vi "test_min-wpts.vi"() -> ()   [LabVIEW 2019]
uses:
  Ctrl/waypoint_buf.ctl
panel:
  in  "Tab Control":enum32{"Page 1", "ref"}(tab)
  out "XY Graph":cluster{cluster{dbl, dbl}[]}[](graph)=[{[{1.0, 2.0}]}, {[{1.0, 3.0}, {1.0980171403295607, 2.995184726672197}, {1.1950903220161282, 2.9807852804032304}, {1.2902846772544623, 2.9569403357322086}, {1.3826834323650898, 2.923879532511287}, {1.4713967368259977, 2.881921264348355}, {1.5555702330196022, 2.8314696123025453}, {1.6343932841636455, 2.773010453362737}, {1.7071067811865475, 2.7071067811865475}, {1.7730104533627369, 2.6343932841636457}, {1.8314696123025453, 2.555570233019602}, {1.881921264348355, 2.471396736825998}, {1.9238795325112867, 2.3826834323650896}, {1.956940335732209, 2.2902846772544625}, {1.9807852804032304, 2.1950903220161284}, {1.9951847266721967, 2.098017140329561}, {2.0, 2.0}, {1.995184726672197, 1.9019828596704393}, {1.9807852804032304, 1.8049096779838718}, {1.956940335732209, 1.709715322745538}, {1.9238795325112867, 1.6173165676349104}, {1.881921264348355, 1.5286032631740023}, {1.8314696123025453, 1.444429766980398}, {1.773010453362737, 1.3656067158363547}, {1.7071067811865475, 1.2928932188134525}, {1.6343932841636455, 1.2269895466372631}, {1.5555702330196022, 1.1685303876974547}, {1.471396736825998, 1.118078735651645}, {1.3826834323650898, 1.0761204674887133}, {1.2902846772544625, 1.0430596642677912}, {1.1950903220161286, 1.0192147195967696}, {1.0980171403295609, 1.0048152733278033}, {1.0000000000000002, 1.0}, {0.9019828596704395, 1.004815273327803}, {0.8049096779838716, 1.0192147195967696}, {0.709715322745538, 1.043059664267791}, {0.6173165676349104, 1.076120467488713}, {0.5286032631740023, 1.118078735651645}, {0.44442976698039804, 1.1685303876974547}, {0.36560671583635473, 1.226989546637263}, {0.29289321881345254, 1.2928932188134523}, {0.22698954663726334, 1.365606715836354}, {0.16853038769745476, 1.4444297669803978}, {0.11807873565164506, 1.528603263174002}, {0.07612046748871348, 1.6173165676349097}, {0.043059664267791176, 1.7097153227455375}, {0.01921471959676968, 1.8049096779838714}, {0.004815273327803071, 1.9019828596704396}, {0.0, 1.9999999999999998}, {0.004815273327803071, 2.09801714032956}, {0.01921471959676957, 2.1950903220161284}, {0.043059664267791065, 2.290284677254462}, {0.07612046748871337, 2.38268343236509}, {0.11807873565164495, 2.4713967368259975}, {0.16853038769745454, 2.5555702330196017}, {0.22698954663726312, 2.6343932841636457}, {0.2928932188134523, 2.7071067811865475}, {0.36560671583635407, 2.773010453362737}, {0.4444297669803978, 2.8314696123025453}, {0.5286032631740021, 2.881921264348355}, {0.6173165676349096, 2.9238795325112865}, {0.7097153227455375, 2.9569403357322086}, {0.8049096779838713, 2.9807852804032304}, {0.9019828596704395, 2.995184726672197}, {0.9999999999999998, 3.0}]}, {[{-1.0, 1.5}, {3.5, 3.0}, {5.0, 2.5}, {10.0, 4.0}, {13.0, 0.0}, {10.0, -3.0}, {5.0, -4.0}, {2.0, -3.0}, {-1.0, -5.0}, {-2.0, -2.0}, {-1.0, 1.0}]}, {[{-1.0, 1.5}, {-0.9042553191489362, 1.5319148936170213}, {-0.8085106382978724, 1.5638297872340425}, {-0.7127659574468085, 1.5957446808510638}, {-0.6170212765957447, 1.627659574468085}, {-0.5212765957446809, 1.6595744680851063}, {-0.42553191489361697, 1.6914893617021276}, {-0.32978723404255317, 1.7234042553191489}, {-0.23404255319148937, 1.7553191489361701}, {-0.13829787234042556, 1.7872340425531914}, {-0.042553191489361764, 1.8191489361702127}, {0.05319148936170204, 1.851063829787234}, {0.14893617021276606, 1.8829787234042552}, {0.24468085106382986, 1.9148936170212765}, {0.34042553191489366, 1.9468085106382977}, {0.43617021276595747, 1.978723404255319}, {0.5319148936170213, 2.0106382978723403}, {0.6276595744680851, 2.0425531914893615}, {0.7234042553191489, 2.074468085106383}, {0.8191489361702127, 2.106382978723404}, {0.9148936170212765, 2.1382978723404253}, {1.0106382978723403, 2.1702127659574466}, {1.106382978723404, 2.202127659574468}, {1.2021276595744679, 2.234042553191489}, {1.2978723404255321, 2.2659574468085104}, {1.393617021276596, 2.297872340425532}, {1.4893617021276597, 2.329787234042553}, {1.5851063829787235, 2.3617021276595747}, {1.6808510638297873, 2.3936170212765955}, {1.7765957446808511, 2.425531914893617}, {1.872340425531915, 2.457446808510638}, {1.9680851063829787, 2.4893617021276597}, {2.0638297872340425, 2.5212765957446805}, {2.1595744680851063, 2.5531914893617023}, {2.25531914893617, 2.585106382978723}, {2.351063829787234, 2.617021276595745}, {2.4468085106382977, 2.6489361702127656}, {2.5425531914893615, 2.6808510638297873}, {2.6382978723404253, 2.712765957446808}, {2.734042553191489, 2.74468085106383}, {2.829787234042553, 2.7765957446808507}, {2.925531914893617, 2.8085106382978724}, {3.0212765957446805, 2.840425531914893}, {3.117021276595745, 2.872340425531915}, {3.212765957446808, 2.9042553191489358}, {3.3085106382978724, 2.9361702127659575}, {3.4042553191489358, 2.9680851063829783}, {3.5, 3.0}, {3.59375, 2.96875}, {3.6875, 2.9375}, {3.78125, 2.90625}, {3.875, 2.875}, {3.96875, 2.84375}, {4.0625, 2.8125}, {4.15625, 2.78125}, {4.25, 2.75}, {4.34375, 2.71875}, {4.4375, 2.6875}, {4.53125, 2.65625}, {4.625, 2.625}, {4.71875, 2.59375}, {4.8125, 2.5625}, {4.90625, 2.53125}, {5.0, 2.5}, {5.096153846153846, 2.5288461538461537}, {5.1923076923076925, 2.5576923076923075}, {5.288461538461538, 2.5865384615384617}, {5.384615384615385, 2.6153846153846154}, {5.480769230769231, 2.644230769230769}, {5.576923076923077, 2.673076923076923}, {5.673076923076923, 2.701923076923077}, {5.769230769230769, 2.730769230769231}, {5.865384615384615, 2.7596153846153846}, {5.961538461538462, 2.7884615384615383}, {6.0576923076923075, 2.8173076923076925}, {6.153846153846154, 2.8461538461538463}, {6.25, 2.875}, {6.346153846153847, 2.9038461538461537}, {6.4423076923076925, 2.9326923076923075}, {6.538461538461538, 2.9615384615384617}, {6.634615384615385, 2.9903846153846154}, {6.730769230769231, 3.019230769230769}, {6.826923076923077, 3.0480769230769234}, {6.923076923076923, 3.076923076923077}, {7.019230769230769, 3.105769230769231}, {7.115384615384615, 3.1346153846153846}, {7.211538461538462, 3.1634615384615383}, {7.307692307692308, 3.1923076923076925}, {7.403846153846154, 3.2211538461538463}, {7.5, 3.25}, {7.596153846153847, 3.2788461538461537}, {7.6923076923076925, 3.3076923076923075}, {7.788461538461538, 3.3365384615384617}, {7.884615384615385, 3.3653846153846154}, {7.980769230769231, 3.394230769230769}, {8.076923076923077, 3.4230769230769234}, {8.173076923076923, 3.451923076923077}, {8.26923076923077, 3.480769230769231}, {8.365384615384615, 3.5096153846153846}, {8.461538461538462, 3.5384615384615383}, {8.557692307692308, 3.5673076923076925}, {8.653846153846153, 3.5961538461538463}, {8.75, 3.625}, {8.846153846153847, 3.653846153846154}, {8.942307692307693, 3.6826923076923075}, {9.038461538461538, 3.7115384615384617}, {9.134615384615385, 3.7403846153846154}, {9.23076923076923, 3.769230769230769}, {9.326923076923077, 3.7980769230769234}, {9.423076923076923, 3.826923076923077}, {9.51923076923077, 3.855769230769231}, {9.615384615384617, 3.8846153846153846}, {9.711538461538462, 3.9134615384615383}, {9.807692307692308, 3.9423076923076925}, {9.903846153846153, 3.9711538461538463}, {10.0, 4.0}, {10.06, 3.92}, {10.12, 3.84}, {10.18, 3.76}, {10.24, 3.68}, {10.3, 3.6}, {10.36, 3.52}, {10.42, 3.44}, {10.48, 3.36}, {10.54, 3.2800000000000002}, {10.6, 3.2}, {10.66, 3.12}, {10.72, 3.04}, {10.78, 2.96}, {10.84, 2.88}, {10.9, 2.8}, {10.96, 2.7199999999999998}, {11.02, 2.6399999999999997}, {11.08, 2.56}, {11.14, 2.48}, {11.2, 2.4}, {11.26, 2.3200000000000003}, {11.32, 2.24}, {11.379999999999999, 2.16}, {11.44, 2.08}, {11.5, 2.0}, {11.56, 1.92}, {11.62, 1.8399999999999999}, {11.68, 1.7599999999999998}, {11.74, 1.6800000000000002}, {11.8, 1.6}, {11.86, 1.52}, {11.92, 1.44}, {11.98, 1.3599999999999999}, {12.04, 1.2799999999999998}, {12.1, 1.1999999999999997}, {12.16, 1.12}, {12.219999999999999, 1.04}, {12.28, 0.96}, {12.34, 0.8799999999999999}, {12.4, 0.7999999999999998}, {12.46, 0.7199999999999998}, {12.52, 0.6400000000000001}, {12.58, 0.56}, {12.64, 0.48}, {12.7, 0.3999999999999999}, {12.76, 0.31999999999999984}, {12.82, 0.23999999999999977}, {12.879999999999999, 0.16000000000000014}, {12.94, 0.08000000000000007}, {13.0, 0.0}, {12.928571428571429, -0.07142857142857142}, {12.857142857142858, -0.14285714285714285}, {12.785714285714286, -0.21428571428571427}, {12.714285714285714, -0.2857142857142857}, {12.642857142857142, -0.3571428571428571}, {12.571428571428571, -0.42857142857142855}, {12.5, -0.5}, {12.428571428571429, -0.5714285714285714}, {12.357142857142858, -0.6428571428571428}, {12.285714285714286, -0.7142857142857142}, {12.214285714285714, -0.7857142857142857}, {12.142857142857142, -0.8571428571428571}, {12.071428571428571, -0.9285714285714285}, {12.0, -1.0}, {11.928571428571429, -1.0714285714285714}, {11.857142857142858, -1.1428571428571428}, {11.785714285714286, -1.2142857142857142}, {11.714285714285715, -1.2857142857142856}, {11.642857142857142, -1.357142857142857}, {11.571428571428571, -1.4285714285714284}, {11.5, -1.5}, {11.428571428571429, -1.5714285714285714}, {11.357142857142858, -1.6428571428571428}, {11.285714285714286, -1.7142857142857142}, {11.214285714285715, -1.7857142857142856}, {11.142857142857142, -1.857142857142857}, {11.071428571428571, -1.9285714285714284}, {11.0, -2.0}, {10.928571428571429, -2.071428571428571}, {10.857142857142858, -2.142857142857143}, {10.785714285714286, -2.214285714285714}, {10.714285714285715, -2.2857142857142856}, {10.642857142857142, -2.357142857142857}, {10.571428571428571, -2.4285714285714284}, {10.5, -2.5}, {10.428571428571429, -2.571428571428571}, {10.357142857142858, -2.642857142857143}, {10.285714285714286, -2.714285714285714}, {10.214285714285715, -2.7857142857142856}, {10.142857142857142, -2.8571428571428568}, {10.071428571428571, -2.9285714285714284}, {10.0, -3.0}, {9.901960784313726, -3.019607843137255}, {9.803921568627452, -3.0392156862745097}, {9.705882352941176, -3.0588235294117645}, {9.607843137254902, -3.0784313725490198}, {9.509803921568627, -3.0980392156862746}, {9.411764705882353, -3.1176470588235294}, {9.313725490196079, -3.1372549019607843}, {9.215686274509803, -3.156862745098039}, {9.117647058823529, -3.176470588235294}, {9.019607843137255, -3.196078431372549}, {8.92156862745098, -3.215686274509804}, {8.823529411764707, -3.235294117647059}, {8.725490196078432, -3.2549019607843137}, {8.627450980392156, -3.2745098039215685}, {8.529411764705882, -3.2941176470588234}, {8.431372549019608, -3.313725490196078}, {8.333333333333334, -3.3333333333333335}, {8.235294117647058, -3.3529411764705883}, {8.137254901960784, -3.372549019607843}, {8.03921568627451, -3.392156862745098}, {7.9411764705882355, -3.411764705882353}, {7.843137254901961, -3.431372549019608}, {7.745098039215686, -3.450980392156863}, {7.647058823529411, -3.4705882352941178}, {7.549019607843137, -3.4901960784313726}, {7.450980392156863, -3.5098039215686274}, {7.352941176470589, -3.5294117647058822}, {7.254901960784314, -3.549019607843137}, {7.156862745098039, -3.568627450980392}, {7.0588235294117645, -3.588235294117647}, {6.96078431372549, -3.607843137254902}, {6.862745098039216, -3.627450980392157}, {6.764705882352941, -3.6470588235294117}, {6.666666666666666, -3.6666666666666665}, {6.568627450980392, -3.686274509803922}, {6.470588235294118, -3.7058823529411766}, {6.372549019607844, -3.7254901960784315}, {6.2745098039215685, -3.7450980392156863}, {6.176470588235294, -3.764705882352941}, {6.078431372549019, -3.784313725490196}, {5.980392156862745, -3.803921568627451}, {5.882352941176471, -3.8235294117647056}, {5.784313725490196, -3.843137254901961}, {5.686274509803922, -3.8627450980392157}, {5.588235294117647, -3.8823529411764706}, {5.490196078431373, -3.9019607843137254}, {5.392156862745098, -3.9215686274509802}, {5.294117647058823, -3.9411764705882355}, {5.196078431372549, -3.9607843137254903}, {5.098039215686274, -3.980392156862745}, {5.0, -4.0}, {4.90625, -3.96875}, {4.8125, -3.9375}, {4.71875, -3.90625}, {4.625, -3.875}, {4.53125, -3.84375}, {4.4375, -3.8125}, {4.34375, -3.78125}, {4.25, -3.75}, {4.15625, -3.71875}, {4.0625, -3.6875}, {3.96875, -3.65625}, {3.875, -3.625}, {3.78125, -3.59375}, {3.6875, -3.5625}, {3.59375, -3.53125}, {3.5, -3.5}, {3.40625, -3.46875}, {3.3125, -3.4375}, {3.21875, -3.40625}, {3.125, -3.375}, {3.03125, -3.34375}, {2.9375, -3.3125}, {2.84375, -3.28125}, {2.75, -3.25}, {2.65625, -3.21875}, {2.5625, -3.1875}, {2.46875, -3.15625}, {2.375, -3.125}, {2.28125, -3.09375}, {2.1875, -3.0625}, {2.09375, -3.03125}, {2.0, -3.0}, {1.9166666666666667, -3.0555555555555554}, {1.8333333333333333, -3.111111111111111}, {1.75, -3.1666666666666665}, {1.6666666666666667, -3.2222222222222223}, {1.5833333333333335, -3.2777777777777777}, {1.5, -3.3333333333333335}, {1.4166666666666667, -3.388888888888889}, {1.3333333333333335, -3.4444444444444446}, {1.25, -3.5}, {1.1666666666666667, -3.5555555555555554}, {1.0833333333333335, -3.611111111111111}, {1.0, -3.6666666666666665}, {0.9166666666666667, -3.7222222222222223}, {0.8333333333333335, -3.7777777777777777}, {0.75, -3.833333333333333}, {0.6666666666666667, -3.888888888888889}, {0.5833333333333335, -3.9444444444444446}, {0.5, -4.0}, {0.41666666666666674, -4.055555555555555}, {0.3333333333333335, -4.111111111111111}, {0.25, -4.166666666666666}, {0.16666666666666674, -4.222222222222222}, {0.08333333333333348, -4.277777777777778}, {0.0, -4.333333333333333}, {-0.08333333333333304, -4.388888888888889}, {-0.16666666666666652, -4.444444444444445}, {-0.25, -4.5}, {-0.33333333333333304, -4.555555555555555}, {-0.4166666666666665, -4.611111111111111}, {-0.5, -4.666666666666666}, {-0.583333333333333, -4.722222222222222}, {-0.6666666666666665, -4.777777777777778}, {-0.75, -4.833333333333333}, {-0.833333333333333, -4.888888888888889}, {-0.9166666666666665, -4.944444444444445}, {-1.0, -5.0}, {-1.03125, -4.90625}, {-1.0625, -4.8125}, {-1.09375, -4.71875}, {-1.125, -4.625}, {-1.15625, -4.53125}, {-1.1875, -4.4375}, {-1.21875, -4.34375}, {-1.25, -4.25}, {-1.28125, -4.15625}, {-1.3125, -4.0625}, {-1.34375, -3.96875}, {-1.375, -3.875}, {-1.40625, -3.78125}, {-1.4375, -3.6875}, {-1.46875, -3.59375}, {-1.5, -3.5}, {-1.53125, -3.40625}, {-1.5625, -3.3125}, {-1.59375, -3.21875}, {-1.625, -3.125}, {-1.65625, -3.03125}, {-1.6875, -2.9375}, {-1.71875, -2.84375}, {-1.75, -2.75}, {-1.78125, -2.65625}, {-1.8125, -2.5625}, {-1.84375, -2.46875}, {-1.875, -2.375}, {-1.90625, -2.28125}, {-1.9375, -2.1875}, {-1.96875, -2.09375}, {-2.0, -2.0}, {-1.96875, -1.90625}, {-1.9375, -1.8125}, {-1.90625, -1.71875}, {-1.875, -1.625}, {-1.84375, -1.53125}, {-1.8125, -1.4375}, {-1.78125, -1.34375}, {-1.75, -1.25}, {-1.71875, -1.15625}, {-1.6875, -1.0625}, {-1.65625, -0.96875}, {-1.625, -0.875}, {-1.59375, -0.78125}, {-1.5625, -0.6875}, {-1.53125, -0.59375}, {-1.5, -0.5}, {-1.46875, -0.40625}, {-1.4375, -0.3125}, {-1.40625, -0.21875}, {-1.375, -0.125}, {-1.34375, -0.03125}, {-1.3125, 0.0625}, {-1.28125, 0.15625}, {-1.25, 0.25}, {-1.21875, 0.34375}, {-1.1875, 0.4375}, {-1.15625, 0.53125}, {-1.125, 0.625}, {-1.09375, 0.71875}, {-1.0625, 0.8125}, {-1.03125, 0.90625}]}]
  in  "way point":cluster{dbl, dbl}[](array[cluster])=[{-1.0, 1.5}, {3.5, 3.0}, {5.0, 2.5}, {10.0, 4.0}, {13.0, 0.0}, {10.0, -3.0}, {5.0, -4.0}, {2.0, -3.0}, {-1.0, -5.0}, {-2.0, -2.0}, {-1.0, 1.0}]
  in  "agv":cluster{dbl, dbl}={1.0, 2.0} {"?" scale=-5.0..15.0; "?" scale=-5.0..10.0}
  in  "lookahed cfg in":T1={"lookahead pt n"=64.0, "lookahead distance "=2.0}
  out "looktail":cluster{"x":dbl, "y":dbl} {"x" format="%.2f"; "y" format="%.2f"}
  out "lookahead":cluster{"x":dbl, "y":dbl} {"x" format="%.2f"; "y" format="%.2f"}
  in  "stop":bool
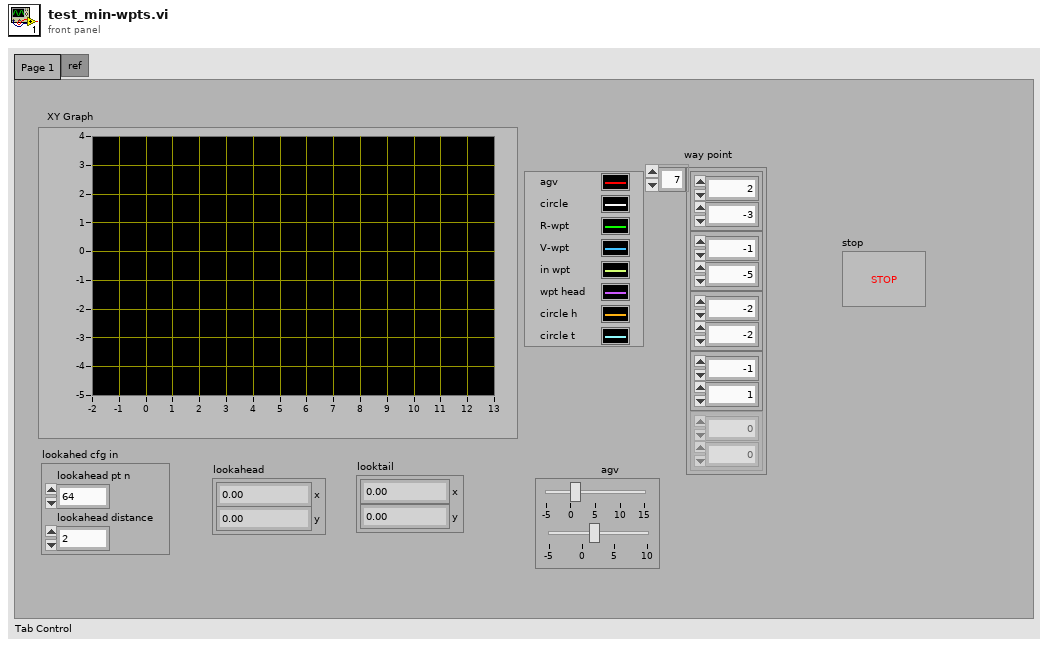
[diagram p1: front panel]
types:
  T1 = cluster{"lookahead pt n":dbl, "lookahead distance ":dbl}
  T2 = typedef "waypoint_buf.ctl" = enum16{"clear", "write", "read"}
  T3 = cluster{"lookahead pt n":dbl, "lookahead distance":dbl}
  T4 = cluster{"incircle wpt":cluster{dbl, dbl}[], "lookahead":cluster{"x":dbl, "y":dbl}, "looktail":cluster{"x":dbl, "y":dbl}, "agv incircle":cluster{dbl, dbl}[]}
  T5 = cluster{"waypoint out":cluster{"x":dbl, "y":dbl}[]}
  T6 = cluster{"waypoint out":cluster{"x":dbl, "y":dbl}[]}[]
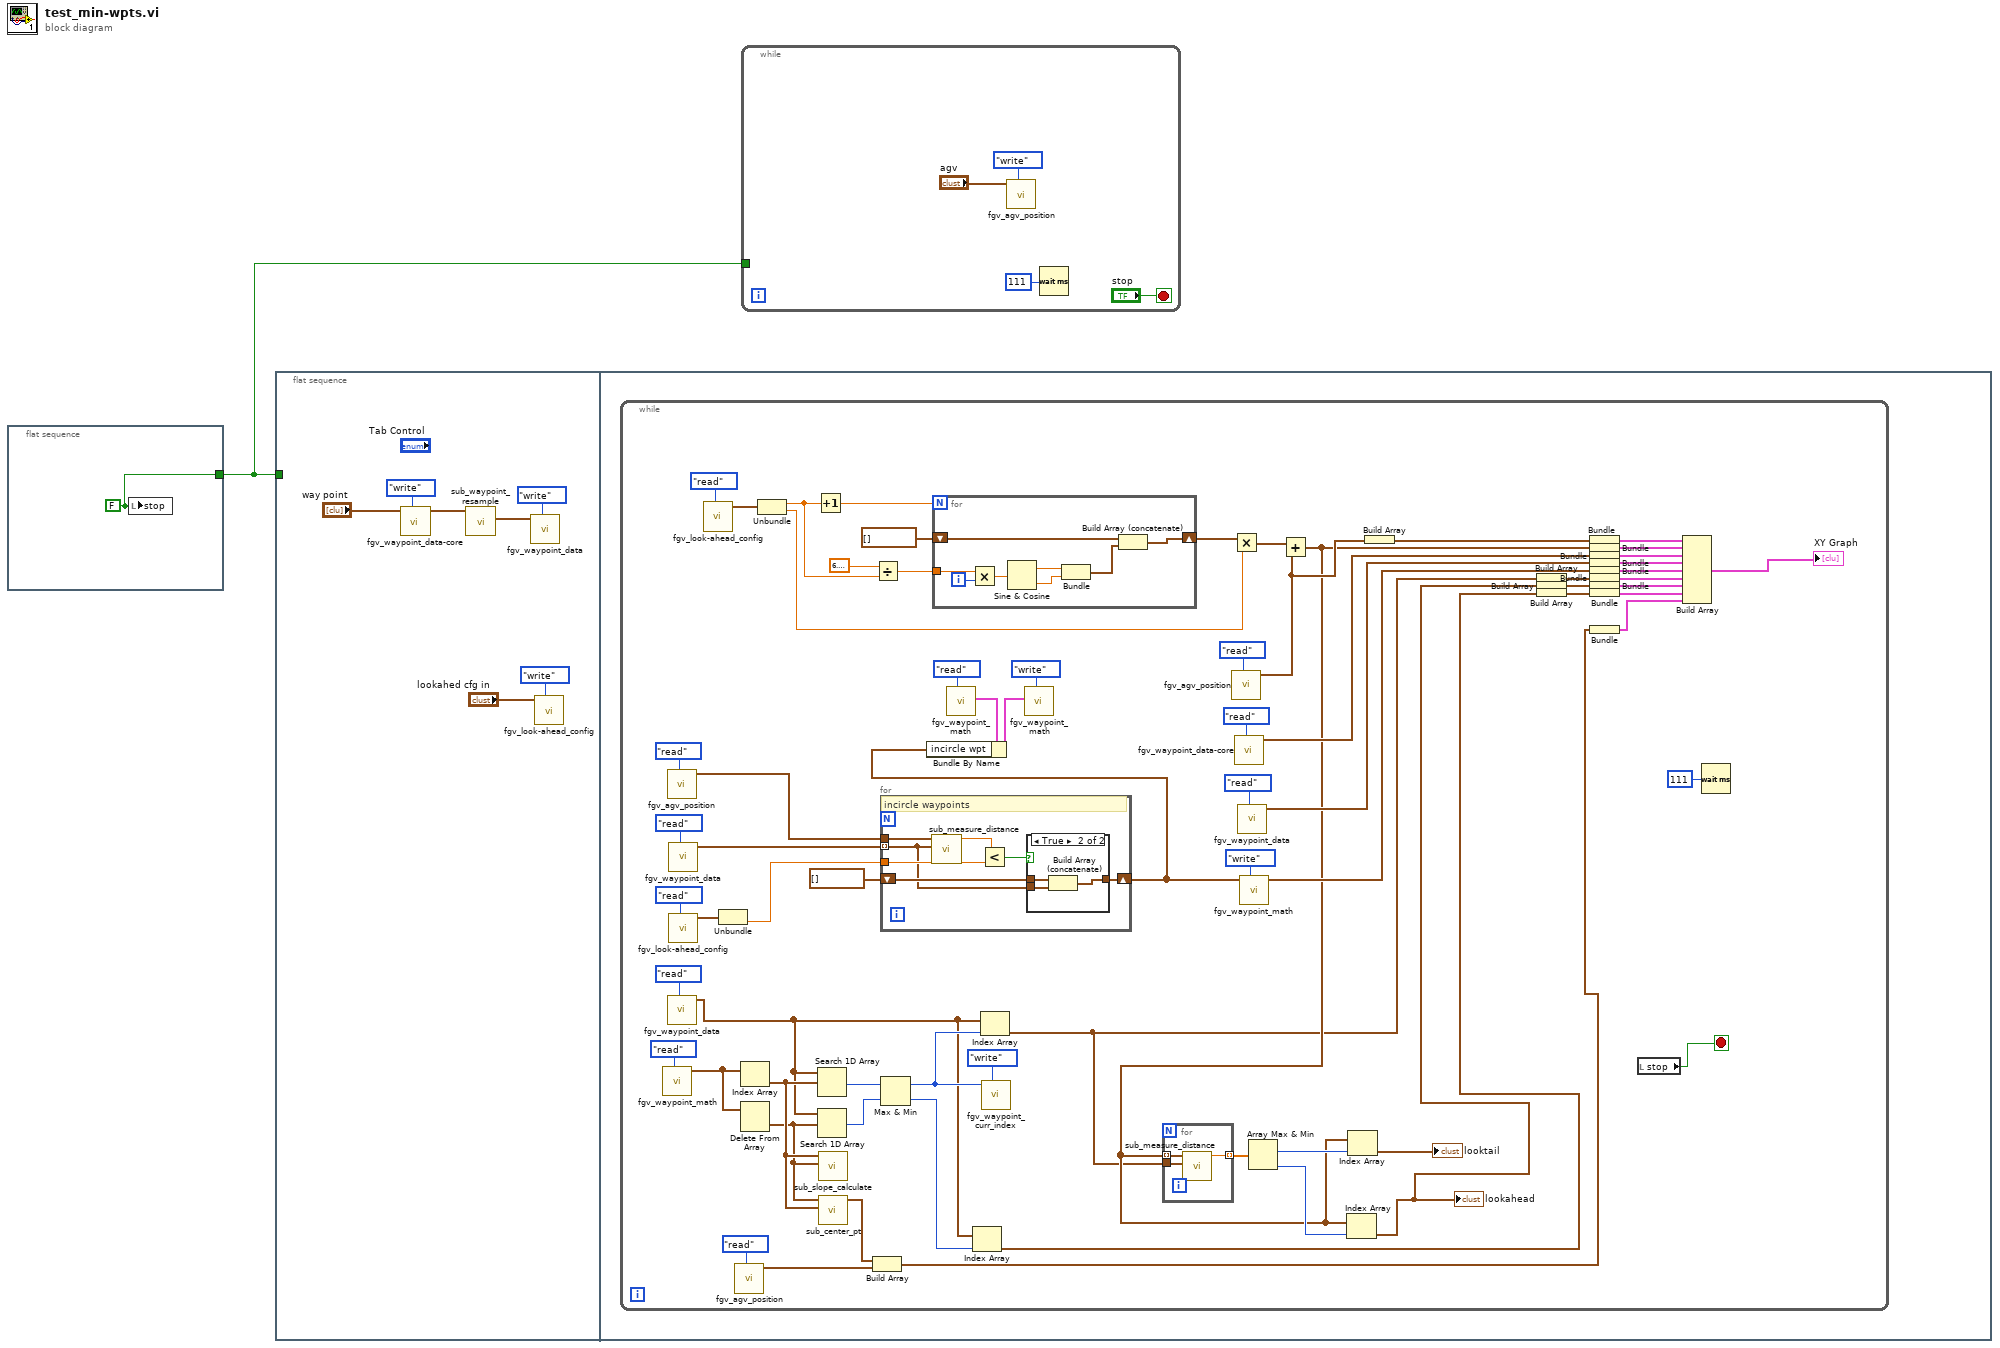
[diagram p0: block diagram]
diagram:
  n1 = flat-sequence {
    tunnel: [w2] -> w1
    frame #0 {
      w2 = FALSE ("stop")
      n2 = local write "stop"(w2) -> ()
    }
  }
  n3 = flat-sequence {
    tunnel: w1 -> [_]
    frame #0 {
      n4 = call "fgv_waypoint_data-core.vi"("cmd"=waypoint_buf."write", "ori-waypoint"="way point") -> ("waypoint out"=w3:cluster{"x":dbl, "y":dbl}[])  [unwired: 9 in]
      n5 = call "sub_waypoint_resample.vi"("line point"=w3) -> ("interpolate 1d array"=w6:cluster{dbl, dbl}[])  [unwired: 9 in, 1 out]
      n6 = call "fgv_waypoint_data.vi"("cmd"=waypoint_buf."write", "waypoint in"=w6) -> ()  [unwired: 7 in, 3 out]
      n7 = call "fgv_look-ahead_config.vi"("cmd"=enum16{"read", "write"}."write", "lookahed cfg in"="lookahed cfg in") -> ()  [unwired: 9 in, 1 out]
    }
    frame #1 {
      n8 = while {
        stop <- w25 stop-if-true
        n9 = call "fgv_waypoint_math.vi"("cmd"=waypoint_buf."read") -> ("waypoint out"=w29:cluster{"x":dbl, "y":dbl}[])  [unwired: 9 in, 1 out]
        n10 = call "fgv_agv_position.vi"("cmd"=enum16{"write", "read"}."read") -> ("agv curr utm out"=w57:cluster{dbl, dbl})  [unwired: 8 in, 2 out]
        n11 = call "fgv_waypoint_data.vi"("cmd"=waypoint_buf."read") -> ("waypoint out"=w17:cluster{"x":dbl, "y":dbl}[])  [unwired: 8 in, 2 out]
        n12 = call "fgv_waypoint_data.vi"("cmd"=waypoint_buf."read") -> ("waypoint out"=w16:cluster{"x":dbl, "y":dbl}[])  [unwired: 8 in, 2 out]
        n13 = call "fgv_look-ahead_config.vi"("cmd"=enum16{"read", "write"}."read") -> ("lookahed cfg out"=w55:T3)  [unwired: 10 in]
        n14 = call "fgv_look-ahead_config.vi"("cmd"=enum16{"read", "write"}."read") -> ("lookahed cfg out"=w66:T3)  [unwired: 10 in]
        n15 = Unbundle(w55) -> ("lookahead distance"=w54:dbl)  [unwired: 1 out]
        n16 = call "fgv_agv_position.vi"("cmd"=enum16{"write", "read"}."read") -> ("agv curr utm out"=w20:cluster{dbl, dbl})  [unwired: 8 in, 2 out]
        n17 = Index Array(array=w29) -> (element=w48:cluster{"x":dbl, "y":dbl})  [unwired: 1 in]
        n18 = Delete From Array(array=w29) -> (deleted portion=w47:cluster{"x":dbl, "y":dbl})  [unwired: 2 in, 1 out]
        n19 = Unbundle(w66) -> ("lookahead pt n"=w65:dbl, "lookahead distance"=w64:dbl)
        n20 = Increment(x=w65) -> (x+1=w74:dbl)
        n21 = Search 1D Array(1D array=w17, element=w48) -> (index of element=w43:i32)  [unwired: 1 in]
        n22 = Search 1D Array(1D array=w17, element=w47) -> (index of element=w44:i32)  [unwired: 1 in]
        n23 = call "sub_slope_calculate.vi"("point n+1"=w47, "point n"=w48) -> ()  [unwired: 7 in, 3 out]
        n24 = call "sub_center_pt.vi"("point-2"=w48, "point-1"=w47) -> ("center"=w21:cluster{"x":dbl, "y":dbl})  [unwired: 9 in]
        n25 = Build Array(w21, w20) -> (w19:cluster{"x":dbl, "y":dbl}[])
        n26 = Divide(x=6.283185307179586, y=w65) -> (x/y=w78:dbl)
        n27 = for {
          tunnel: w16 -> [w84] mode=indexing
          tunnel: w57 -> [w89]
          shift-right: [w83] -> w11
          shift-left: cluster{"x":dbl, "y":dbl}[] [] -> [w86]
          tunnel: w54 -> [w87]
          # "incircle waypoints"
          n28 = call "sub_measure_distance.vi"("pt 2"=w84, "pt 1"=w89) -> ("distance"=w88:dbl)  [unwired: 9 in]
          n29 = Less?(x=w88, y=w87) -> (x < y?=w85:bool)
          n30 = case shown="True" w85 {
            tunnel: w86 -> [w90 w93]
            tunnel: w84 -> [_ w92]
            tunnel: [w90 w91] -> w83
            frame False {
            }
            frame True {
              n31 = Build Array (concatenate)(w93, w92) -> (w91:cluster{"x":dbl, "y":dbl}[])
            }
          }
        }
        n32 = Max & Min(x=w43, y=w44) -> (max(x,y)=w46:i32, min(x,y)=w45:i32)
        n33 = for {
          N: w74 -> [_]
          tunnel: w78 -> [w97]
          shift-right: [w99] -> w61
          shift-left: cluster{dbl, dbl}[] [] -> [w98]
          i -> [w96]
          n34 = Multiply(x=w97, y=w96) -> (x*y=w95:dbl)
          n35 = Sine & Cosine(0:w95) -> (1:w100:dbl, 2:w101:dbl)
          n36 = Bundle(w100, w101) -> (w94:cluster{dbl, dbl})  [unwired: 1 in]
          n37 = Build Array (concatenate)(w98, w94) -> (w99:cluster{dbl, dbl}[])
        }
        n38 = call "fgv_waypoint_math.vi"("cmd"=waypoint_buf."read") -> ("Cluster 2"=w13:T4)  [unwired: 9 in, 1 out]
        n39 = Bundle By Name(cluster=w13, "incircle wpt"=w11) -> (w12:T4)
        n40 = Index Array(array=w17, index=w45) -> (element=w34:cluster{"x":dbl, "y":dbl})
        n41 = Index Array(array=w17, index=w46) -> (element=w33:cluster{"x":dbl, "y":dbl})
        n42 = call "fgv_waypoint_curr_index.vi"("cmd"=enum16{"write", "read"}."write", "index in"=w46) -> ()  [unwired: 9 in, 1 out]
        n43 = call "fgv_waypoint_math.vi"("cmd"=waypoint_buf."write", "Cluster"=w12) -> ()  [unwired: 8 in, 2 out]
        n44 = Multiply(x=w61, y=w64) -> (x*y=w63:cluster{dbl, dbl}[])
        n45 = call "fgv_agv_position.vi"("cmd"=enum16{"write", "read"}."read") -> ("agv curr utm out"=w62:cluster{dbl, dbl})  [unwired: 8 in, 2 out]
        n46 = call "fgv_waypoint_data-core.vi"("cmd"=waypoint_buf."read") -> ("waypoint out"=w49:cluster{"x":dbl, "y":dbl}[])  [unwired: 10 in]
        n47 = call "fgv_waypoint_data.vi"("cmd"=waypoint_buf."read") -> ("waypoint out"=w60:cluster{"x":dbl, "y":dbl}[])  [unwired: 8 in, 2 out]
        n48 = call "fgv_waypoint_math.vi"("cmd"=waypoint_buf."write", "incircle wpt"=w11) -> ("waypoint out"=w51:cluster{"x":dbl, "y":dbl}[])  [unwired: 8 in, 1 out]
        n49 = Add(x=w63, y=w62) -> (x+y=w38:cluster{dbl, dbl}[])
        n50 = for {
          tunnel: w38 -> [w82] mode=indexing
          tunnel: w33 -> [w81]
          tunnel: [w80] -> w39 mode=indexing
          n51 = call "sub_measure_distance.vi"("pt 2"=w81, "pt 1"=w82) -> ("distance"=w80:dbl)  [unwired: 9 in]
        }
        n52 = Array Max & Min(array=w39) -> (max index (indices)=w41:i32, min index (indices)=w40:i32)  [unwired: 2 out]
        n53 = Index Array(array=w38, index=w40) -> (element=w32:cluster{dbl, dbl})
        "lookahead" <- w32
        n54 = Index Array(array=w38, index=w41) -> (element=→"looktail":cluster{dbl, dbl})
        n55 = Build Array(w62) -> (w70:cluster{dbl, dbl}[])
        n56 = Build Array(w33) -> (w37:cluster{"x":dbl, "y":dbl}[])
        n57 = Build Array(w32) -> (w36:cluster{dbl, dbl}[])
        n58 = Build Array(w34) -> (w35:cluster{"x":dbl, "y":dbl}[])
        n59 = Bundle(w70) -> (w71:cluster{cluster{dbl, dbl}[]})  [unwired: 1 in]
        n60 = Bundle(w38) -> (w77:cluster{cluster{dbl, dbl}[]})  [unwired: 1 in]
        n61 = Bundle("waypoint out"=w49) -> (w75:T5)  [unwired: 1 in]
        n62 = Bundle("waypoint out"=w60) -> (w72:T5)  [unwired: 1 in]
        n63 = Bundle("waypoint out"=w51) -> (w53:T5)  [unwired: 1 in]
        n64 = Bundle(w37) -> (w28:cluster{cluster{"x":dbl, "y":dbl}[]})  [unwired: 1 in]
        n65 = Bundle(w36) -> (w26:cluster{cluster{dbl, dbl}[]})  [unwired: 1 in]
        n66 = Bundle(w35) -> (w27:cluster{cluster{"x":dbl, "y":dbl}[]})  [unwired: 1 in]
        n67 = Bundle(w19) -> (w23:cluster{cluster{"x":dbl, "y":dbl}[]})  [unwired: 1 in]
        n68 = local read "stop"() -> (w25:bool)
        n69 = Build Array(w71, w77, w75, w72, w53, w28, w26, w27, w23) -> (→"XY Graph":T6)
        n70 = Wait (ms)(milliseconds to wait=u32 111) -> ()  [unwired: 1 out]
      }
    }
  }
  n71 = while {
    tunnel: w1 -> [_]
    stop <- "stop" stop-if-true
    n72 = call "fgv_agv_position.vi"("cmd"=enum16{"write", "read"}."write", "agv curr utm in"="agv") -> ()  [unwired: 7 in, 3 out]
    n73 = Wait (ms)(milliseconds to wait=u32 111) -> ()  [unwired: 1 out]
  }
